vi "Refresh HH Listbox.vi"(8 "Command":T1[](array[typedef])=[{"Mode"=enum."Off", "Digital Input"=enum."Unused", "Polarity"=FALSE, "Frequency [Hz]"=0.0, "Duty Cycle [%]"=0.0, "TDC Offset [CAD]"=0.0, "Window Start [DBTDC]"=0.0, "Window End [DBTDC]"=0.0, "Angles"=[{"Enable"=FALSE, "Location [DBTDC]"=0.0, "Duration [s]"=0.0}, {"Enable"=FALSE, "Location [DBTDC]"=0.0, "Duration [s]"=0.0}, {"Enable"=FALSE, "Location [DBTDC]"=0.0, "Duration [s]"=0.0}, {"Enable"=FALSE, "Location [DBTDC]"=0.0, "Duration [s]"=0.0}], "Skip Fire"=FALSE, "Skip Fire Index"=0}, {"Mode"=enum."Off", "Digital Input"=enum."Unused", "Polarity"=FALSE, "Frequency [Hz]"=0.0, "Duty Cycle [%]"=0.0, "TDC Offset [CAD]"=0.0, "Window Start [DBTDC]"=0.0, "Window End [DBTDC]"=0.0, "Angles"=[{"Enable"=FALSE, "Location [DBTDC]"=0.0, "Duration [s]"=0.0}, {"Enable"=FALSE, "Location [DBTDC]"=0.0, "Duration [s]"=0.0}, {"Enable"=FALSE, "Location [DBTDC]"=0.0, "Duration [s]"=0.0}, {"Enable"=FALSE, "Location [DBTDC]"=0.0, "Duration [s]"=0.0}], "Skip Fire"=FALSE, "Skip Fire Index"=0}, {"Mode"=enum."Off", "Digital Input"=enum."Unused", "Polarity"=FALSE, "Frequency [Hz]"=0.0, "Duty Cycle [%]"=0.0, "TDC Offset [CAD]"=0.0, "Window Start [DBTDC]"=0.0, "Window End [DBTDC]"=0.0, "Angles"=[{"Enable"=FALSE, "Location [DBTDC]"=0.0, "Duration [s]"=0.0}, {"Enable"=FALSE, "Location [DBTDC]"=0.0, "Duration [s]"=0.0}, {"Enable"=FALSE, "Location [DBTDC]"=0.0, "Duration [s]"=0.0}, {"Enable"=FALSE, "Location [DBTDC]"=0.0, "Duration [s]"=0.0}], "Skip Fire"=FALSE, "Skip Fire Index"=0}, {"Mode"=enum."Off", "Digital Input"=enum."Unused", "Polarity"=FALSE, "Frequency [Hz]"=0.0, "Duty Cycle [%]"=0.0, "TDC Offset [CAD]"=0.0, "Window Start [DBTDC]"=0.0, "Window End [DBTDC]"=0.0, "Angles"=[{"Enable"=FALSE, "Location [DBTDC]"=0.0, "Duration [s]"=0.0}, {"Enable"=FALSE, "Location [DBTDC]"=0.0, "Duration [s]"=0.0}, {"Enable"=FALSE, "Location [DBTDC]"=0.0, "Duration [s]"=0.0}, {"Enable"=FALSE, "Location [DBTDC]"=0.0, "Duration [s]"=0.0}], "Skip Fire"=FALSE, "Skip Fire Index"=0}, {"Mode"=enum."Off", "Digital Input"=enum."Unused", "Polarity"=FALSE, "Frequency [Hz]"=0.0, "Duty Cycle [%]"=0.0, "TDC Offset [CAD]"=0.0, "Window Start [DBTDC]"=0.0, "Window End [DBTDC]"=0.0, "Angles"=[{"Enable"=FALSE, "Location [DBTDC]"=0.0, "Duration [s]"=0.0}, {"Enable"=FALSE, "Location [DBTDC]"=0.0, "Duration [s]"=0.0}, {"Enable"=FALSE, "Location [DBTDC]"=0.0, "Duration [s]"=0.0}, {"Enable"=FALSE, "Location [DBTDC]"=0.0, "Duration [s]"=0.0}], "Skip Fire"=FALSE, "Skip Fire Index"=0}, {"Mode"=enum."Off", "Digital Input"=enum."Unused", "Polarity"=FALSE, "Frequency [Hz]"=0.0, "Duty Cycle [%]"=0.0, "TDC Offset [CAD]"=0.0, "Window Start [DBTDC]"=0.0, "Window End [DBTDC]"=0.0, "Angles"=[{"Enable"=FALSE, "Location [DBTDC]"=0.0, "Duration [s]"=0.0}, {"Enable"=FALSE, "Location [DBTDC]"=0.0, "Duration [s]"=0.0}, {"Enable"=FALSE, "Location [DBTDC]"=0.0, "Duration [s]"=0.0}, {"Enable"=FALSE, "Location [DBTDC]"=0.0, "Duration [s]"=0.0}], "Skip Fire"=FALSE, "Skip Fire Index"=0}, {"Mode"=enum."Off", "Digital Input"=enum."Unused", "Polarity"=FALSE, "Frequency [Hz]"=0.0, "Duty Cycle [%]"=0.0, "TDC Offset [CAD]"=0.0, "Window Start [DBTDC]"=0.0, "Window End [DBTDC]"=0.0, "Angles"=[{"Enable"=FALSE, "Location [DBTDC]"=0.0, "Duration [s]"=0.0}, {"Enable"=FALSE, "Location [DBTDC]"=0.0, "Duration [s]"=0.0}, {"Enable"=FALSE, "Location [DBTDC]"=0.0, "Duration [s]"=0.0}, {"Enable"=FALSE, "Location [DBTDC]"=0.0, "Duration [s]"=0.0}], "Skip Fire"=FALSE, "Skip Fire Index"=0}, {"Mode"=enum."Off", "Digital Input"=enum."Unused", "Polarity"=FALSE, "Frequency [Hz]"=0.0, "Duty Cycle [%]"=0.0, "TDC Offset [CAD]"=0.0, "Window Start [DBTDC]"=0.0, "Window End [DBTDC]"=0.0, "Angles"=[{"Enable"=FALSE, "Location [DBTDC]"=0.0, "Duration [s]"=0.0}, {"Enable"=FALSE, "Location [DBTDC]"=0.0, "Duration [s]"=0.0}, {"Enable"=FALSE, "Location [DBTDC]"=0.0, "Duration [s]"=0.0}, {"Enable"=FALSE, "Location [DBTDC]"=0.0, "Duration [s]"=0.0}], "Skip Fire"=FALSE, "Skip Fire Index"=0}] {"Skip Fire Index" max=7; "Angles"."Duration [s]" format="%#_3p"; "Frequency [Hz]" format="%#_3p"}, 9 "Names":string[](array[string]), 10 "Config":T5[](array[typedef]) {"ISeq"."Duration [s]" min=0 max=26 format="%#_3p"; "ISeq"."Lower [A]" min=0 max=8 format="%#_3p"; "ISeq"."Upper [A]" min=0 max=8 format="%#_3p"}, 11 "_Listbox":refnum<vi>) -> (0 "Command out":T1[](array[typedef])=[{"Mode"=enum."Off", "Digital Input"=enum."Unused", "Polarity"=FALSE, "Frequency [Hz]"=0.0, "Duty Cycle [%]"=0.0, "TDC Offset [CAD]"=0.0, "Window Start [DBTDC]"=0.0, "Window End [DBTDC]"=0.0, "Angles"=[{"Enable"=FALSE, "Location [DBTDC]"=0.0, "Duration [s]"=0.0}, {"Enable"=FALSE, "Location [DBTDC]"=0.0, "Duration [s]"=0.0}, {"Enable"=FALSE, "Location [DBTDC]"=0.0, "Duration [s]"=0.0}, {"Enable"=FALSE, "Location [DBTDC]"=0.0, "Duration [s]"=0.0}], "Skip Fire"=FALSE, "Skip Fire Index"=0}, {"Mode"=enum."Off", "Digital Input"=enum."Unused", "Polarity"=FALSE, "Frequency [Hz]"=0.0, "Duty Cycle [%]"=0.0, "TDC Offset [CAD]"=0.0, "Window Start [DBTDC]"=0.0, "Window End [DBTDC]"=0.0, "Angles"=[{"Enable"=FALSE, "Location [DBTDC]"=0.0, "Duration [s]"=0.0}, {"Enable"=FALSE, "Location [DBTDC]"=0.0, "Duration [s]"=0.0}, {"Enable"=FALSE, "Location [DBTDC]"=0.0, "Duration [s]"=0.0}, {"Enable"=FALSE, "Location [DBTDC]"=0.0, "Duration [s]"=0.0}], "Skip Fire"=FALSE, "Skip Fire Index"=0}, {"Mode"=enum."Off", "Digital Input"=enum."Unused", "Polarity"=FALSE, "Frequency [Hz]"=0.0, "Duty Cycle [%]"=0.0, "TDC Offset [CAD]"=0.0, "Window Start [DBTDC]"=0.0, "Window End [DBTDC]"=0.0, "Angles"=[{"Enable"=FALSE, "Location [DBTDC]"=0.0, "Duration [s]"=0.0}, {"Enable"=FALSE, "Location [DBTDC]"=0.0, "Duration [s]"=0.0}, {"Enable"=FALSE, "Location [DBTDC]"=0.0, "Duration [s]"=0.0}, {"Enable"=FALSE, "Location [DBTDC]"=0.0, "Duration [s]"=0.0}], "Skip Fire"=FALSE, "Skip Fire Index"=0}, {"Mode"=enum."Off", "Digital Input"=enum."Unused", "Polarity"=FALSE, "Frequency [Hz]"=0.0, "Duty Cycle [%]"=0.0, "TDC Offset [CAD]"=0.0, "Window Start [DBTDC]"=0.0, "Window End [DBTDC]"=0.0, "Angles"=[{"Enable"=FALSE, "Location [DBTDC]"=0.0, "Duration [s]"=0.0}, {"Enable"=FALSE, "Location [DBTDC]"=0.0, "Duration [s]"=0.0}, {"Enable"=FALSE, "Location [DBTDC]"=0.0, "Duration [s]"=0.0}, {"Enable"=FALSE, "Location [DBTDC]"=0.0, "Duration [s]"=0.0}], "Skip Fire"=FALSE, "Skip Fire Index"=0}, {"Mode"=enum."Off", "Digital Input"=enum."Unused", "Polarity"=FALSE, "Frequency [Hz]"=0.0, "Duty Cycle [%]"=0.0, "TDC Offset [CAD]"=0.0, "Window Start [DBTDC]"=0.0, "Window End [DBTDC]"=0.0, "Angles"=[{"Enable"=FALSE, "Location [DBTDC]"=0.0, "Duration [s]"=0.0}, {"Enable"=FALSE, "Location [DBTDC]"=0.0, "Duration [s]"=0.0}, {"Enable"=FALSE, "Location [DBTDC]"=0.0, "Duration [s]"=0.0}, {"Enable"=FALSE, "Location [DBTDC]"=0.0, "Duration [s]"=0.0}], "Skip Fire"=FALSE, "Skip Fire Index"=0}, {"Mode"=enum."Off", "Digital Input"=enum."Unused", "Polarity"=FALSE, "Frequency [Hz]"=0.0, "Duty Cycle [%]"=0.0, "TDC Offset [CAD]"=0.0, "Window Start [DBTDC]"=0.0, "Window End [DBTDC]"=0.0, "Angles"=[{"Enable"=FALSE, "Location [DBTDC]"=0.0, "Duration [s]"=0.0}, {"Enable"=FALSE, "Location [DBTDC]"=0.0, "Duration [s]"=0.0}, {"Enable"=FALSE, "Location [DBTDC]"=0.0, "Duration [s]"=0.0}, {"Enable"=FALSE, "Location [DBTDC]"=0.0, "Duration [s]"=0.0}], "Skip Fire"=FALSE, "Skip Fire Index"=0}, {"Mode"=enum."Off", "Digital Input"=enum."Unused", "Polarity"=FALSE, "Frequency [Hz]"=0.0, "Duty Cycle [%]"=0.0, "TDC Offset [CAD]"=0.0, "Window Start [DBTDC]"=0.0, "Window End [DBTDC]"=0.0, "Angles"=[{"Enable"=FALSE, "Location [DBTDC]"=0.0, "Duration [s]"=0.0}, {"Enable"=FALSE, "Location [DBTDC]"=0.0, "Duration [s]"=0.0}, {"Enable"=FALSE, "Location [DBTDC]"=0.0, "Duration [s]"=0.0}, {"Enable"=FALSE, "Location [DBTDC]"=0.0, "Duration [s]"=0.0}], "Skip Fire"=FALSE, "Skip Fire Index"=0}, {"Mode"=enum."Off", "Digital Input"=enum."Unused", "Polarity"=FALSE, "Frequency [Hz]"=0.0, "Duty Cycle [%]"=0.0, "TDC Offset [CAD]"=0.0, "Window Start [DBTDC]"=0.0, "Window End [DBTDC]"=0.0, "Angles"=[{"Enable"=FALSE, "Location [DBTDC]"=0.0, "Duration [s]"=0.0}, {"Enable"=FALSE, "Location [DBTDC]"=0.0, "Duration [s]"=0.0}, {"Enable"=FALSE, "Location [DBTDC]"=0.0, "Duration [s]"=0.0}, {"Enable"=FALSE, "Location [DBTDC]"=0.0, "Duration [s]"=0.0}], "Skip Fire"=FALSE, "Skip Fire Index"=0}] {"Skip Fire Index" max=7; "Angles"."Duration [s]" format="%#_3p"; "Frequency [Hz]" format="%#_3p"}, 2 "Config out":T5[](array[typedef]) {"ISeq"."Duration [s]" min=0 max=26 format="%#_3p"; "ISeq"."Lower [A]" min=0 max=8 format="%#_3p"; "ISeq"."Upper [A]" min=0 max=8 format="%#_3p"})   [LabVIEW 2016, in "DCM System Explorer.lvlib"]
uses:
  DCM System Explorer.lvlib
  <vilib>/Powertrain Controls/Device Drivers/DCM/HH/RT/Config.ctl
  <vilib>/Powertrain Controls/Device Drivers/DCM/HH/RT/Mode.ctl
  <vilib>/Powertrain Controls/Device Drivers/DCM/HH/RT/ISeq.ctl
  <vilib>/Powertrain Controls/Device Drivers/DCM/HH/RT/Setup.ctl
  <vilib>/Powertrain Controls/Device Drivers/DCM/HH/FPGA/Mode.ctl
  <vilib>/Powertrain Controls/Device Drivers/DCM/Rev0/FPGA/Digital Channel.ctl
  <vilib>/Powertrain Controls/Device Drivers/DCM/HH/RT/Angle Control.ctl
  <vilib>/Powertrain Controls/Device Drivers/DCM/HH/RT/DCM - RT - HH.lvlib
  <vilib>/Powertrain Controls/Device Drivers/DCM/HH/FPGA/DCM - FPGA - HH.lvlib
  <vilib>/Powertrain Controls/Device Drivers/DCM/Rev0/FPGA/DCM - FPGA.lvlib
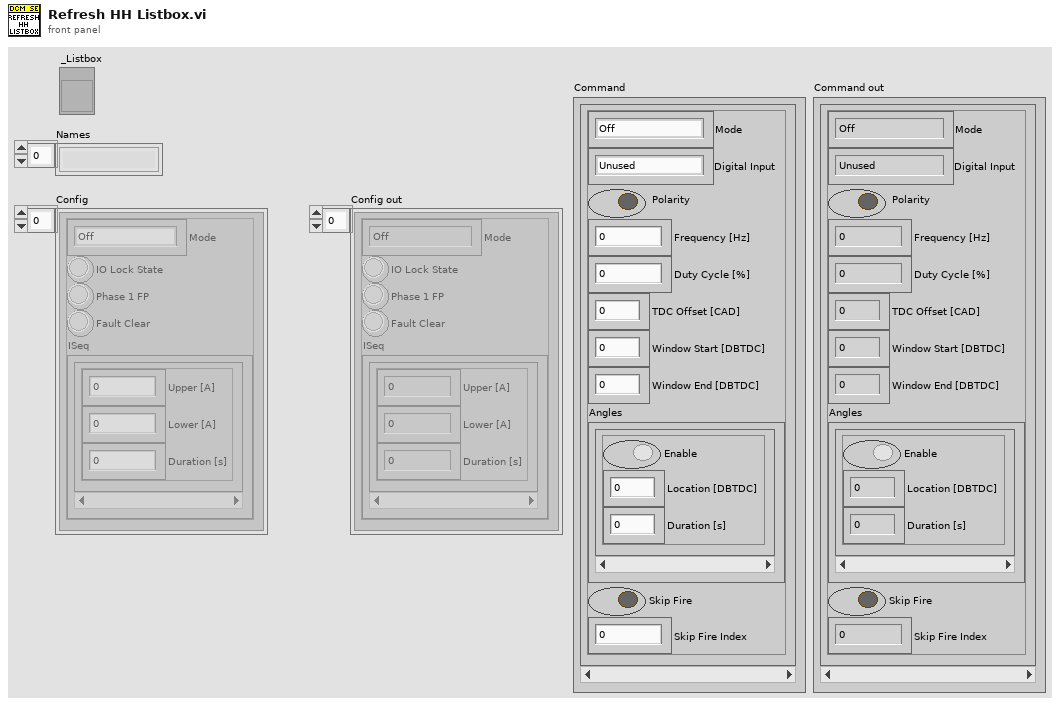
[diagram p1: front panel]
types:
  T1 = typedef "DCM - RT - HH.lvlib/Setup.ctl" = cluster{"Mode":T2, "Digital Input":T3, "Polarity":bool, "Frequency [Hz]":sgl, "Duty Cycle [%]":sgl, "TDC Offset [CAD]":sgl, "Window Start [DBTDC]":sgl, "Window End [DBTDC]":sgl, "Angles":T4[], "Skip Fire":bool, "Skip Fire Index":u8}
  T2 = typedef "DCM - FPGA - HH.lvlib/Mode.ctl" = enum8{"Off", "Direct", "Pulse Width Modulation", "Engine Position Tracking"}
  T3 = typedef "DCM - FPGA.lvlib/Digital Channel.ctl" = enum8{"Unused", "User OS", "Diff IO 1", "Diff IO 2", "Diff IO 3", "Diff IO 4", "Diff IO 5", "Diff IO 6", "Diff IO 7", "Diff IO 8", "Aux 1", "Aux 2", "Aux 3", "Aux 4", "Aux 5", "Aux 6", "Aux 7", "Aux 8", "Aux 9", "Aux 10", "Aux 11", "Aux 12", "Aux 13", "Aux 14", "Aux 15", "Aux 16"}
  T4 = typedef "DCM - RT - HH.lvlib/Angle Control.ctl" = cluster{"Enable":bool, "Location [DBTDC]":sgl, "Duration [s]":sgl}
  T5 = typedef "DCM - RT - HH.lvlib/Config.ctl" = cluster{"Mode":T6, "IO Lock State":bool, "Phase 1 FP":bool, "Fault Clear":bool, "ISeq":T7[]}
  T6 = typedef "DCM - RT - HH.lvlib/Mode.ctl" = enum16{"Off", "Lowside", "Highside", "PFI", "Full H", "3-Phase"}
  T7 = typedef "DCM - RT - HH.lvlib/ISeq.ctl" = cluster{"Upper [A]":sgl, "Lower [A]":sgl, "Duration [s]":sgl}
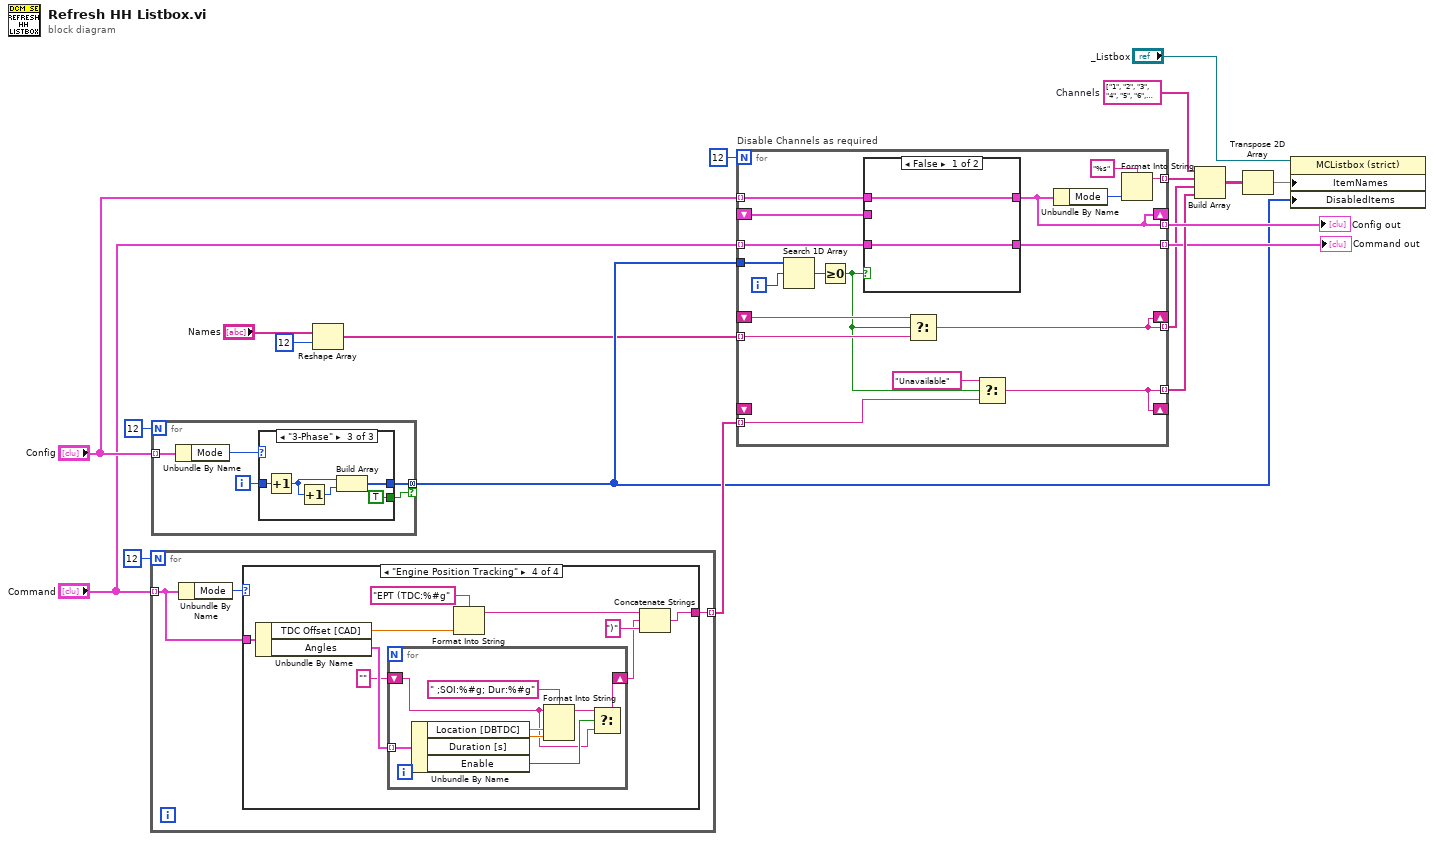
[diagram p0: block diagram]
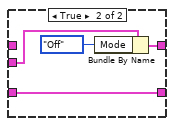
[diagram p2: hidden frame]
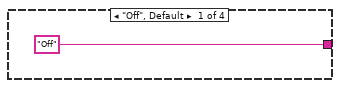
[diagram p3: hidden frame]
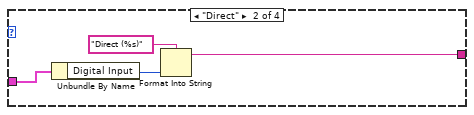
[diagram p4: hidden frame]
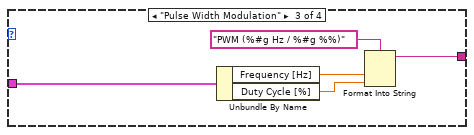
[diagram p5: hidden frame]
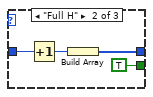
[diagram p7: hidden frame]
diagram:
  w17 = string[] ["1", "2", "3", "4", "5", "6", "7", "8", "9", "10", "11", "12"]  # Channels
  n1 = for {
    N: 12 -> [_]
    tunnel: "Command" -> [w21] mode=indexing
    tunnel: [w20] -> w12 mode=indexing
    n2 = Unbundle By Name(w21) -> ("Mode"=w22:T2)
    n3 = case shown="\"Engine Position Tracking\"" w22 {
      tunnel: w21 -> [_ w27 w32 w40]
      tunnel: ["Off" w24 w28 w36] -> w20
      frame "Off", Default {
      }
      frame "Direct" {
        n4 = Unbundle By Name(w27) -> ("Digital Input"=w25:T3)
        n5 = Format Into String(format string="Direct (%s)", w25) -> (resulting string=w24:string)  [unwired: 2 in, 1 out]
      }
      frame "Pulse Width Modulation" {
        n6 = Unbundle By Name(w32) -> ("Frequency [Hz]"=w30:sgl, "Duty Cycle [%]"=w29:sgl)
        n7 = Format Into String(format string="PWM (%#g Hz / %#g %%)", w30, w29) -> (resulting string=w28:string)  [unwired: 2 in, 1 out]
      }
      frame "Engine Position Tracking" {
        n8 = Unbundle By Name(w40) -> ("TDC Offset [CAD]"=w39:sgl, "Angles"=w38:T4[])
        n9 = for {
          tunnel: w38 -> [w47] mode=indexing
          shift-right: [w43] -> w34
          shift-left: "" -> [w42]
          n10 = Unbundle By Name(w47) -> ("Location [DBTDC]"=w48:sgl, "Duration [s]"=w46:sgl, "Enable"=w45:bool)
          n11 = Format Into String(format string=" ;SOI:%#g; Dur:%#g", initial string=w42, w48, w46) -> (resulting string=w44:string)  [unwired: 1 in, 1 out]
          n12 = Select(t=w44, s=w45, f=w42) -> (s? t:f=w43:string)
        }
        n13 = Format Into String(format string="EPT (TDC:%#g", w39) -> (resulting string=w37:string)  [unwired: 2 in, 1 out]
        n14 = Concatenate Strings(w37, w34, ")" ("string")) -> (w36:string)
      }
    }
  }
  n15 = for {
    N: 12 -> [_]
    tunnel: "Config" -> [w54] mode=indexing
    tunnel: [w51] -> w4 mode=concatenating if=w50
    i -> [w52]
    n16 = Unbundle By Name(w54) -> ("Mode"=w53:T6)
    n17 = case shown="\"3-Phase\"" w53 {
      tunnel: w52 -> [_ w58 w63]
      tunnel: [_ w57 w60] -> w51
      tunnel: [_ TRUE TRUE] -> w50
      frame "Off", Default {
      }
      frame "Full H" {
        n18 = Increment(x=w58) -> (x+1=w56:i32)
        n19 = Build Array(w56) -> (w57:i32[])
      }
      frame "3-Phase" {
        n20 = Increment(x=w63) -> (x+1=w62:i32)
        n21 = Increment(x=w62) -> (x+1=w61:i32)
        n22 = Build Array(w62, w61) -> (w60:i32[])
      }
    }
  }
  n23 = Reshape Array("Names", 12 ("dimension size")) -> (w3:string[])
  n24 = for "Disable Channels as required" {
    N: 12 -> [_]
    tunnel: "Config" -> [w75] mode=indexing
    tunnel: w4 -> [w81]
    tunnel: [w66] -> w13 mode=indexing
    tunnel: [w76] -> w14 mode=indexing
    tunnel: w12 -> [w71] mode=indexing
    tunnel: [w64] -> w11 mode=indexing
    tunnel: [w73] -> w10 mode=indexing
    tunnel: "Command" -> [w74] mode=indexing
    tunnel: w3 -> [w72] mode=indexing
    tunnel: [w70] -> w2 mode=indexing
    shift-right: [w70] -> _
    shift-left: _ -> [w69]
    shift-right: [w64] -> _
    shift-left: _ -> [_]
    shift-right: [w66] -> _
    shift-left: _ -> [w65]
    i -> [w80]
    n25 = Search 1D Array(1D array=w81, element=w80) -> (index of element=w79:i32)  [unwired: 1 in]
    n26 = Greater Or Equal To 0?(x=w79) -> (x >= 0?=w68:bool)
    n27 = case shown="False" w68 {
      tunnel: w75 -> [w83 _]
      tunnel: [w83 w86] -> w66
      tunnel: w74 -> [w82 w87]
      tunnel: [w82 w87] -> w73
      tunnel: w65 -> [_ w84]
      frame False {
      }
      frame True {
        n28 = Bundle By Name(cluster=w84, "Mode"=Mode."Off") -> (w86:T5)
      }
    }
    n29 = Select(t=w69, s=w68, f=w72) -> (s? t:f=w70:string)
    n30 = Select(t="Unavailable", s=w68, f=w71) -> (s? t:f=w64:string)
    n31 = Unbundle By Name(w66) -> ("Mode"=w77:T6)
    n32 = Format Into String(format string="%s", w77) -> (resulting string=w76:string)  [unwired: 2 in, 1 out]
  }
  "Config out" <- w13
  "Command out" <- w10
  n33 = Build Array(w17, w14, w2, w11) -> (w19:string[][])
  n34 = Transpose 2D Array(2D array=w19) -> (transposed array=w16:string[][])
  n35 = property on="Property Node" class="MCListbox (strict)"(reference="_Listbox", "ItemNames"=w16, "DisabledItems"=w4) -> ()  [unwired: 1 in, 2 out]
